vi "子界面-图像预处理.vi"(8 "穿透图":T2(plugin-control)) -> ()   [LabVIEW 2018]
uses:
  <vilib>/vision/NI_Vision_Development_Module.lvlib
panel:
  out "图像分辨率":T1
  in  "stop":bool caption="停止"
  in  "图像预处理":bool
  in  "自定义色彩":bool
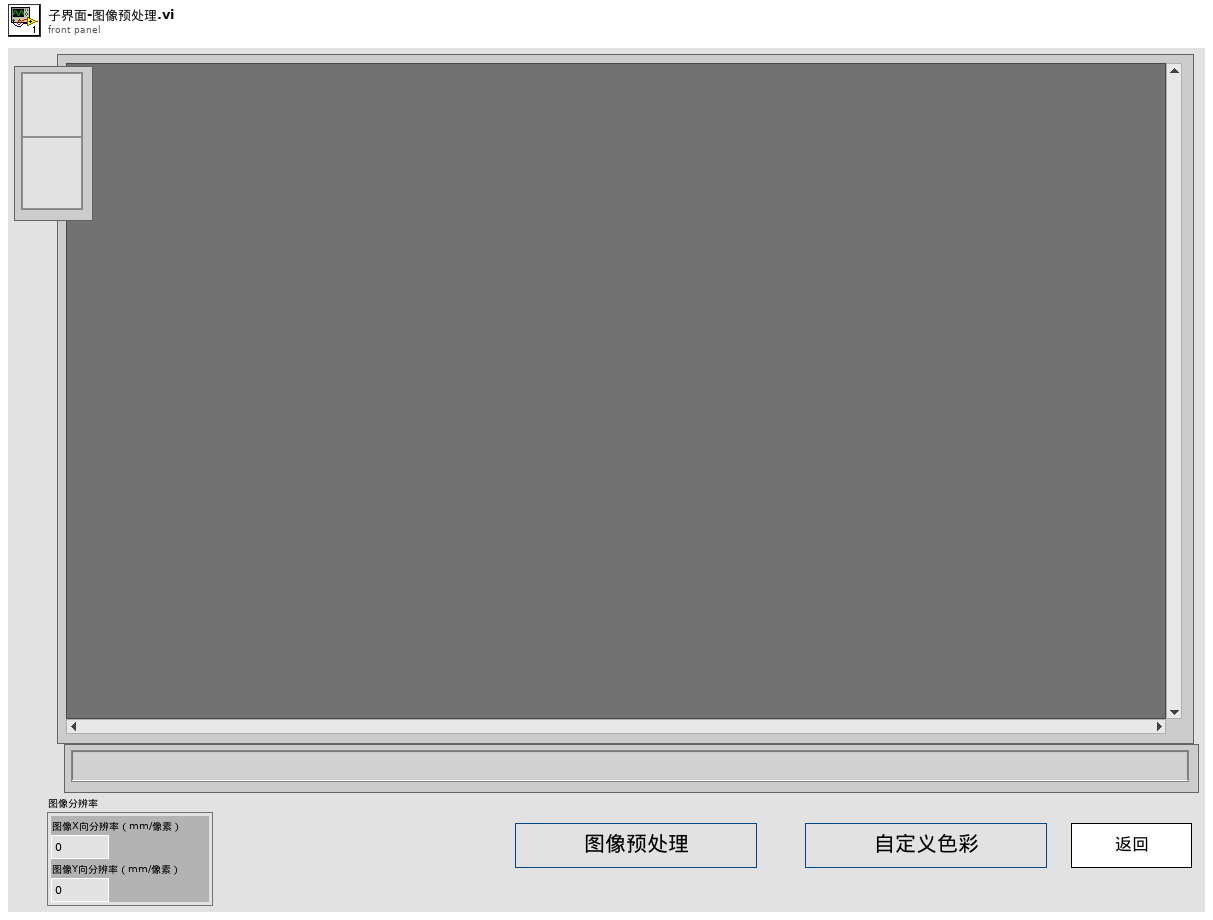
[diagram p1: front panel]
types:
  T1 = cluster{"图像X向分辨率（mm/像素）":dbl, "图像Y向分辨率（mm/像素）":dbl}
  T2 = typedef "IMAQ Image.ctl" = refnum<image>
  T3 = cluster{"Zoom Tool":bool, "Selection Tool":bool, "Pan Tool":bool, "Point Tool":bool, "Line Tool":bool, "Rectangle Tool":bool, "Rotated Rectangle Tool":bool, "Polyline Tool":bool, "Polygon Tool":bool, "Freehand Tool":bool, "Closed Freehand Tool":bool, "Ellipse Tool":bool, "Annulus Tool":bool}
  T4 = enum32{"Linear", "Log", "Exp", "Square", "Square root", "Power X", "Power 1/X"}
  T5 = enum32{"Gray", "Binary", "Gradient", "Rainbow", "Temperature"}
  T6 = enum32{"Invalid", "Standard", "Closed", "Hidden", "Minimized", "Maximized"}
  T7 = cluster{"Red (or Hue) value":u8, "Green (or Sat) value":u8, "Blue (or Light or Val) value":u8}[]
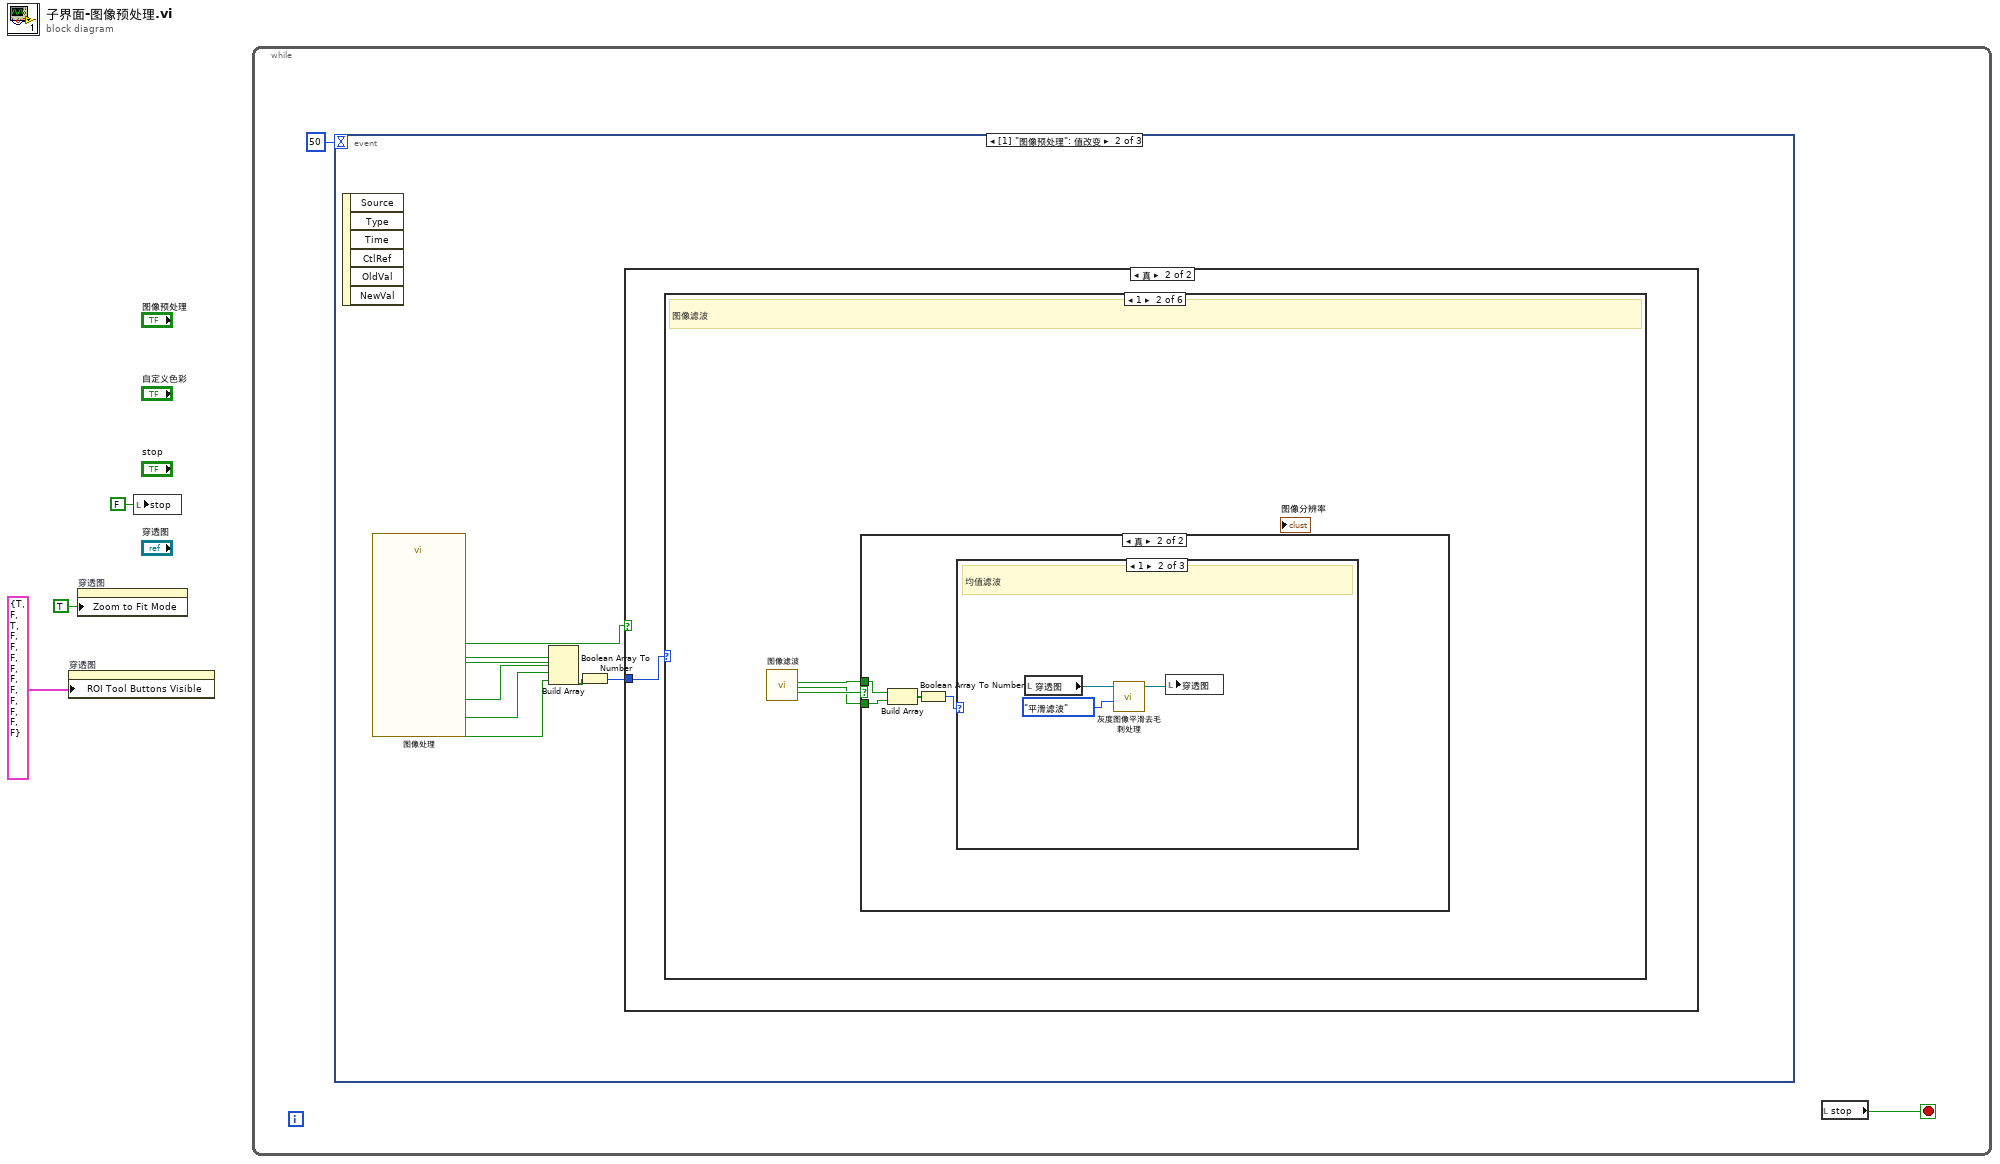
[diagram p0: block diagram]
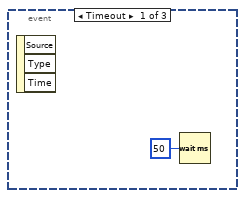
[diagram p2: hidden frame]
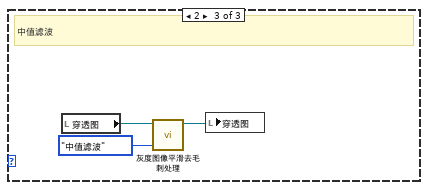
[diagram p7: hidden frame]
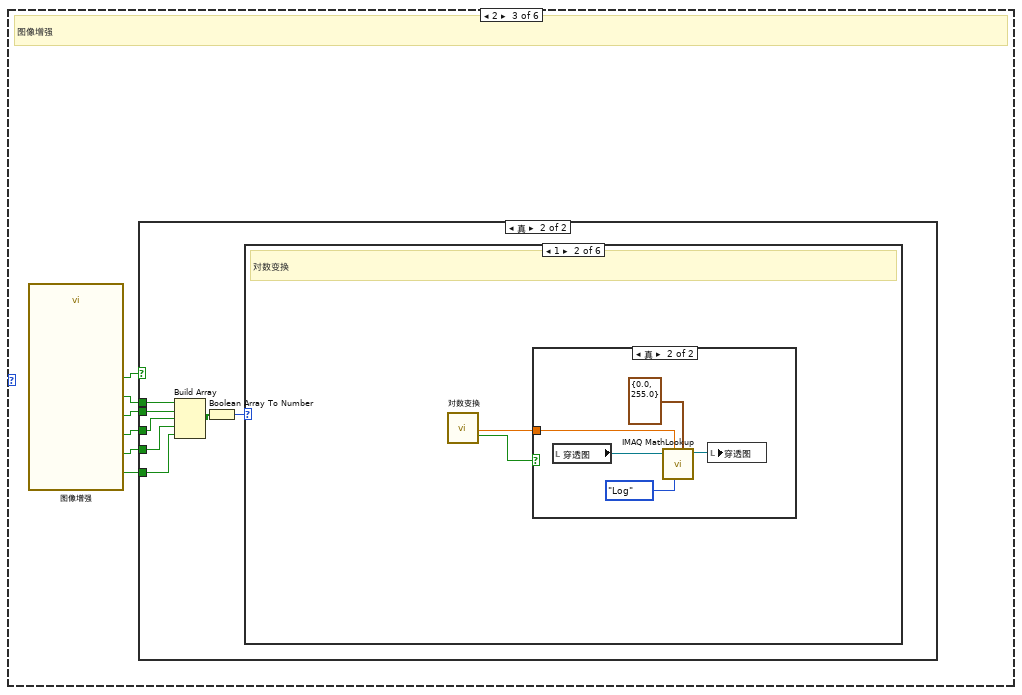
[diagram p8: hidden frame]
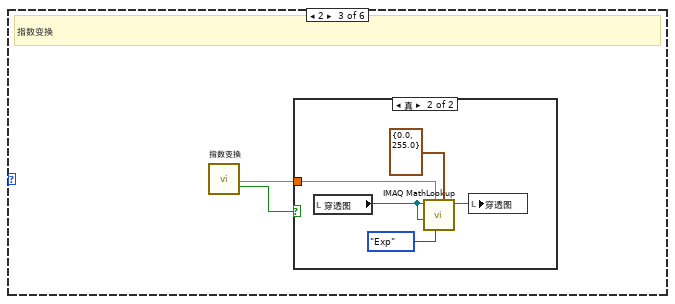
[diagram p12: hidden frame]
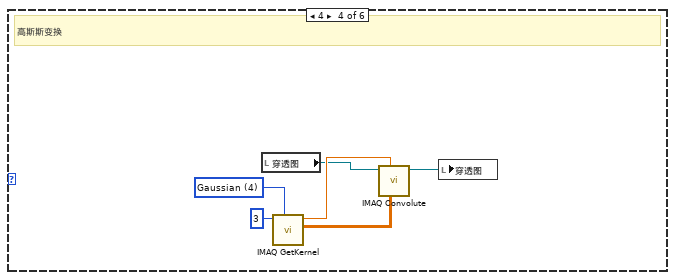
[diagram p14: hidden frame]
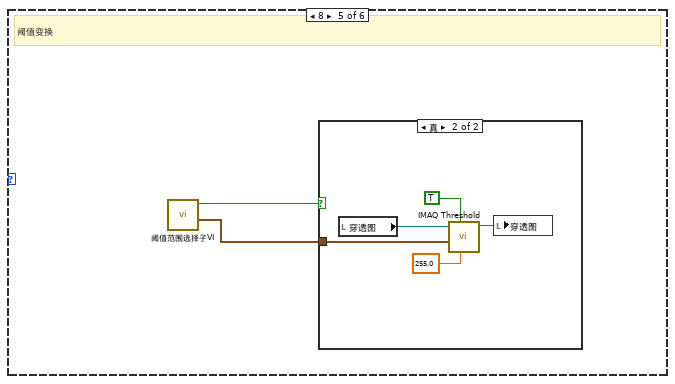
[diagram p15: hidden frame]
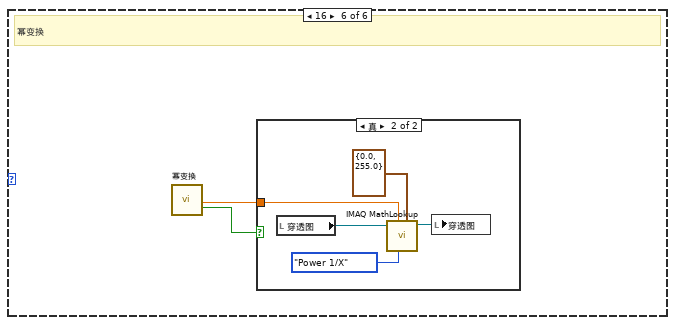
[diagram p17: hidden frame]
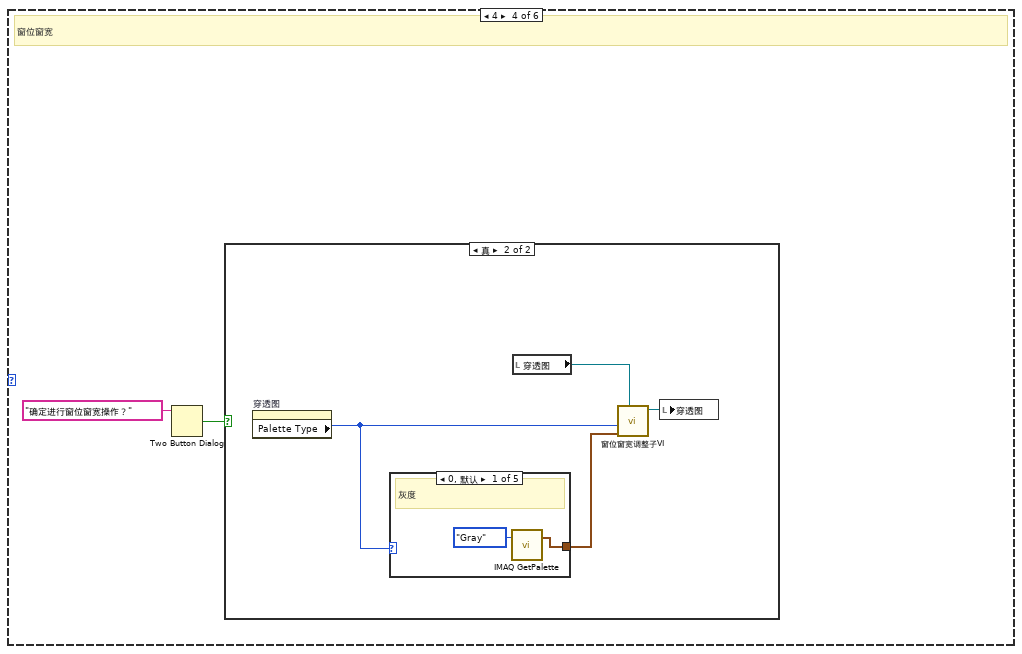
[diagram p19: hidden frame]
diagram:
  n1 = property on="穿透图" class="ImageControl"("ROI Tool Buttons Visible"=T3 {"Zoom Tool"=TRUE, "Selection Tool"=FALSE, "Pan Tool"=TRUE, "Point Tool"=FALSE, "Line Tool"=FALSE, "Rectangle Tool"=FALSE, "Rotated Rectangle Tool"=FALSE, "Polyline Tool"=FALSE, "Polygon Tool"=FALSE, "Freehand Tool"=FALSE, "Closed Freehand Tool"=FALSE, "Ellipse Tool"=FALSE, "Annulus Tool"=FALSE} ("ROI Tool Buttons Visible:All Elements")) -> ()  [unwired: 2 in, 2 out]
  n2 = property on="穿透图" class="ImageControl"("Zoom to Fit Mode"=TRUE) -> ()  [unwired: 2 in, 2 out]
  n3 = local write "stop"(FALSE ("stop")) -> ()
  n4 = while {
    stop <- w5 stop-if-true
    n5 = event shown="[1] \"图像预处理\": 值改变" {
      selector: _ -> [_ _ _]
      dyn-events: _ -> [_ _ _]
      timeout: 50 -> [_ _ _]
      event Timeout {
        n6 = event-data() -> ()  [unwired: 1 in, 3 out]
        n7 = Wait (ms)(milliseconds to wait=u32 50 ("等待时间（毫秒）")) -> ()  [unwired: 1 out]
      }
      event "图像预处理": Value Change {
        n8 = event-data() -> ()  [unwired: 1 in, 6 out]
        n9 = call "图像处理"() -> ("撤销图像处理"=w9:bool, "线性灰度值测量"=w10:bool, "窗位窗宽"=w13:bool, "图像增强"=w11:bool, "图像滤波"=w14:bool, "确定"=w8:bool)  [unwired: 13 in, 1 out]
        n10 = Build Array(w14, w11, w13, w10, w9) -> (w12:bool[])
        n11 = Boolean Array To Number(Boolean array=w12) -> (number=w7:u32)
        n12 = case shown="真" w8 {
          tunnel: w7 -> [_ w15]
          frame False {
          }
          frame True {
            n13 = case shown="1" w15 {
              frame 0, Default {
              }
              frame 1 {
                # "图像滤波"
                n14 = call "图像滤波"() -> ("均值滤波"=w17:bool, "中值滤波"=w16:bool, "确定"=w18:bool)  [unwired: 16 in, 1 out]
                n15 = case shown="真" w18 {
                  tunnel: w17 -> [_ w21]
                  tunnel: w16 -> [_ w20]
                  frame False {
                  }
                  frame True {
                    n16 = Build Array(w21, w20) -> (w22:bool[])
                    n17 = Boolean Array To Number(Boolean array=w22) -> (number=w19:u32)
                    n18 = case shown="1" w19 {
                      frame 0, Default {
                      }
                      frame 1 {
                        # "均值滤波"
                        n19 = local read "穿透图"() -> (w25:T2)
                        n20 = call "灰度图像平滑去毛刺处理.vi"("滤波方法选择"=enum16{"中值滤波", "平滑滤波"}."平滑滤波", "Image"=w25) -> ("Image Out"=w24:T2)  [unwired: 9 in]
                        n21 = local write "穿透图"(w24) -> ()
                      }
                      frame 2 {
                        # "中值滤波"
                        n22 = local read "穿透图"() -> (w28:T2)
                        n23 = call "灰度图像平滑去毛刺处理.vi"("滤波方法选择"=enum16{"中值滤波", "平滑滤波"}."中值滤波", "Image"=w28) -> ("Image Out"=w27:T2)  [unwired: 9 in]
                        n24 = local write "穿透图"(w27) -> ()
                      }
                    }
                  }
                }
              }
              frame 2 {
                # "图像增强"
                n25 = call "图像增强"() -> ("幂变换"=w29:bool, "阈值变换"=w30:bool, "高斯变换"=w31:bool, "指数变换"=w32:bool, "对数变换"=w33:bool, "确定"=w34:bool)  [unwired: 13 in, 1 out]
                n26 = case shown="真" w34 {
                  tunnel: w33 -> [_ w39]
                  tunnel: w32 -> [_ w38]
                  tunnel: w31 -> [_ w37]
                  tunnel: w30 -> [_ w36]
                  tunnel: w29 -> [_ w35]
                  frame False {
                  }
                  frame True {
                    n27 = Build Array(w39, w38, w37, w36, w35) -> (w41:bool[])
                    n28 = Boolean Array To Number(Boolean array=w41) -> (number=w40:u32)
                    n29 = case shown="1" w40 {
                      frame 0, Default {
                      }
                      frame 1 {
                        # "对数变换"
                        n30 = call "对数变换"() -> ("变换系数K"=w42:dbl, "确定"=w43:bool)  [unwired: 17 in, 1 out]
                        n31 = case shown="真" w43 {
                          tunnel: w42 -> [_ w46]
                          frame False {
                          }
                          frame True {
                            n32 = local read "穿透图"() -> (w45:T2)
                            n33 = call "IMAQ MathLookup"("Range"=cluster{"Minimum":sgl, "Maximum":sgl} {"Minimum"=0.0, "Maximum"=255.0}, "Operator"=T4."Log", "X Value"=w46, "Image Src"=w45) -> ("Image Dst Out"=w44:T2)  [unwired: 6 in, 1 out]
                            n34 = local write "穿透图"(w44) -> ()
                          }
                        }
                      }
                      frame 2 {
                        # "指数变换"
                        n35 = call "指数变换"() -> ("变换系数K"=w49:dbl, "确定"=w50:bool)  [unwired: 17 in, 1 out]
                        n36 = case shown="真" w50 {
                          tunnel: w49 -> [_ w51]
                          frame False {
                          }
                          frame True {
                            n37 = local read "穿透图"() -> (w55:T2)
                            n38 = call "IMAQ MathLookup"("Range"=cluster{"Minimum":sgl, "Maximum":sgl} {"Minimum"=0.0, "Maximum"=255.0}, "Operator"=T4."Exp", "X Value"=w51, "Image Dst"=w55, "Image Src"=w55) -> ("Image Dst Out"=w53:T2)  [unwired: 5 in, 1 out]
                            n39 = local write "穿透图"(w53) -> ()
                          }
                        }
                      }
                      frame 4 {
                        w61 = u16 4 items=["Gradient"=1, "Laplacian"=2, "Smoothing"=3, "Gaussian"=4] ("Kernel Family")
                        # "高斯斯变换"
                        n40 = local read "穿透图"() -> (w57:T2)
                        n41 = call "IMAQ GetKernel"("Kernel Family"=w61, "Kernel Size (3,5,...)"=3) -> ("Kernel"=w59:sgl[][], "Divider"=w58:sgl)  [unwired: 6 in, 2 out]
                        n42 = call "IMAQ Convolute"("Kernel"=w59, "Divider (kernel sum)"=w58, "Image Src"=w57) -> ("Image Dst Out"=w56:T2)  [unwired: 7 in, 1 out]
                        n43 = local write "穿透图"(w56) -> ()
                      }
                      frame 8 {
                        # "阈值变换"
                        n44 = call "阈值范围选择子VI.vi"() -> ("阈值范围"=w62:cluster{"Lower value":sgl, "Upper value":sgl}, "确定执行"=w63:bool)  [unwired: 10 in]
                        n45 = case shown="真" w63 {
                          tunnel: w62 -> [_ w67]
                          frame False {
                          }
                          frame True {
                            n46 = local read "穿透图"() -> (w65:T2)
                            n47 = call "IMAQ Threshold"("Replace Value"=sgl 255.0, "Keep/Replace Value (Replace)"=TRUE, "Range"=w67, "Image Src"=w65) -> ("Image Dst Out"=w64:T2)  [unwired: 6 in, 1 out]
                            n48 = local write "穿透图"(w64) -> ()
                          }
                        }
                      }
                      frame 16 {
                        # "幂变换"
                        n49 = call "幂变换"() -> ("变换系数K"=w69:dbl, "确定"=w70:bool)  [unwired: 17 in, 1 out]
                        n50 = case shown="真" w70 {
                          tunnel: w69 -> [_ w73]
                          frame False {
                          }
                          frame True {
                            n51 = local read "穿透图"() -> (w72:T2)
                            n52 = call "IMAQ MathLookup"("Range"=cluster{"Minimum":sgl, "Maximum":sgl} {"Minimum"=0.0, "Maximum"=255.0}, "Operator"=T4."Power 1/X", "X Value"=w73, "Image Src"=w72) -> ("Image Dst Out"=w71:T2)  [unwired: 6 in, 1 out]
                            n53 = local write "穿透图"(w71) -> ()
                          }
                        }
                      }
                    }
                  }
                }
              }
              frame 4 {
                # "窗位窗宽"
                n54 = Two Button Dialog(message="确定进行窗位窗宽操作？" ("消息")) -> (T button?=w77:bool)  [unwired: 2 in]
                n55 = case shown="真" w77 {
                  frame False {
                  }
                  frame True {
                    n56 = property on="穿透图" class="ImageControl"() -> ("Palette Type"=w78:u32)  [unwired: 2 in, 2 out]
                    n57 = case shown="0, 默认" w78 {
                      tunnel: [w82 w84 w86 w88 w90] -> w80
                      frame 0, Default {
                        # "灰度"
                        n58 = call "IMAQ GetPalette"("Palette Number (gray)"=T5."Gray") -> ("Color Palette"=w82:cluster{"Red":u8, "Green":u8, "Blue":u8}[])  [unwired: 4 in, 1 out]
                      }
                      frame 2 {
                        # "梯度"
                        n59 = call "IMAQ GetPalette"("Palette Number (gray)"=T5."Gradient") -> ("Color Palette"=w84:cluster{"Red":u8, "Green":u8, "Blue":u8}[])  [unwired: 4 in, 1 out]
                      }
                      frame 3 {
                        # "彩虹"
                        n60 = call "IMAQ GetPalette"("Palette Number (gray)"=T5."Rainbow") -> ("Color Palette"=w86:cluster{"Red":u8, "Green":u8, "Blue":u8}[])  [unwired: 4 in, 1 out]
                      }
                      frame 4 {
                        # "温度"
                        n61 = call "IMAQ GetPalette"("Palette Number (gray)"=T5."Temperature") -> ("Color Palette"=w88:cluster{"Red":u8, "Green":u8, "Blue":u8}[])  [unwired: 4 in, 1 out]
                      }
                      frame 5 {
                        # "自定义"
                        n62 = property on="穿透图" class="ImageControl"() -> ("User Palette"=w90:cluster{"Red":u8, "Green":u8, "Blue":u8}[])  [unwired: 2 in, 2 out]
                      }
                    }
                    n63 = local read "穿透图"() -> (w79:T2)
                    n64 = call "窗位窗宽调整子VI.vi"("Image in"=w79, "Palette:User Palette"=w80, "Palette:Palette Type"=w78) -> ("Image out"=w81:T2)  [unwired: 8 in]
                    n65 = local write "穿透图"(w81) -> ()
                  }
                }
              }
              frame 8 {
                # "查看线灰度值曲线，用于精确测量"
                n66 = Current VI's Path() -> (path=w97:path)
                n67 = Open VI Reference(vi path=w97) -> (vi reference=w96:refnum<vi>, error out=w94:errorcluster)  [unwired: 5 in]
                n68 = property class="VI"(reference=w96, error in=w94, "FP.State"=T6."Hidden" ("前面板窗口:状态")) -> (reference out=w95:refnum<vi>, error out=w93:errorcluster)
                n69 = Close Reference(reference=w95, error in (no error)=w93) -> (error out=w91:errorcluster)
                n70 = case shown="无错误" w91 {
                  frame No Error {
                    n71 = property on="穿透图" class="ImageControl"() -> ("Palette Type"=w98:u32)  [unwired: 2 in, 2 out]
                    n72 = case shown="5" w98 {
                      tunnel: [w102 w104 w106 w108 w110] -> w100
                      frame 0, Default {
                        # "灰度"
                        n73 = call "IMAQ GetPalette"("Palette Number (gray)"=T5."Gray") -> ("Color Palette"=w102:cluster{"Red":u8, "Green":u8, "Blue":u8}[])  [unwired: 4 in, 1 out]
                      }
                      frame 2 {
                        # "梯度"
                        n74 = call "IMAQ GetPalette"("Palette Number (gray)"=T5."Gradient") -> ("Color Palette"=w104:cluster{"Red":u8, "Green":u8, "Blue":u8}[])  [unwired: 4 in, 1 out]
                      }
                      frame 3 {
                        # "彩虹"
                        n75 = call "IMAQ GetPalette"("Palette Number (gray)"=T5."Rainbow") -> ("Color Palette"=w106:cluster{"Red":u8, "Green":u8, "Blue":u8}[])  [unwired: 4 in, 1 out]
                      }
                      frame 4 {
                        # "温度"
                        n76 = call "IMAQ GetPalette"("Palette Number (gray)"=T5."Temperature") -> ("Color Palette"=w108:cluster{"Red":u8, "Green":u8, "Blue":u8}[])  [unwired: 4 in, 1 out]
                      }
                      frame 5 {
                        # "自定义"
                        n77 = property on="穿透图" class="ImageControl"() -> ("User Palette"=w110:cluster{"Red":u8, "Green":u8, "Blue":u8}[])  [unwired: 2 in, 2 out]
                      }
                    }
                    n78 = local read "穿透图"() -> (w99:T2)
                    n79 = local read "图像分辨率"() -> (w101:T1)
                    n80 = call "线性灰度值曲线查看子VI.vi"("Palette:User Palette"=w100, "图像分辨率"=w101, "Image"=w99) -> ()  [unwired: 9 in]
                  }
                  frame Error {
                  }
                }
              }
              frame 16 {
                # "撤销图像处理，恢复原图"
                n81 = call "IMAQ Create"("Image Name"="P1") -> ("New Image"=w111:T2)  [unwired: 4 in, 1 out]
                n82 = local write "穿透图"(w111) -> ()
              }
            }
          }
        }
      }
      event "自定义色彩": Value Change {
        n83 = event-data() -> ()  [unwired: 1 in, 6 out]
        n84 = call "调色板"() -> ("自定义显示"=w118:bool, "温度显示"=w117:bool, "彩虹显示"=w116:bool, "梯度显示"=w115:bool, "灰度显示"=w114:bool, "确定"=w113:bool)  [unwired: 13 in, 1 out]
        n85 = Build Array(w114, w115, w116, w117, w118) -> (w119:bool[])
        n86 = case shown="真" w113 {
          tunnel: w119 -> [_ w122]
          frame False {
          }
          frame True {
            n87 = Boolean Array To Number(Boolean array=w122) -> (number=w121:u32)
            n88 = case shown="16" w121 {
              tunnel: [w123 w124 w125 w126 w127 w129] -> w120
              frame 0, Default {
                w123 = u32 0 items=["Grayscale", "Binary", "Gradient", "Rainbow", "Temperature", "User Defined", "Binary 16 Bit", "Gradient 16 Bit", "Rainbow 16 Bit", "Temperature 16 Bit", "User Defined 16 Bit"] ("Palette:Palette Type")
              }
              frame 1 {
                w124 = u32 0 items=["Grayscale", "Binary", "Gradient", "Rainbow", "Temperature", "User Defined", "Binary 16 Bit", "Gradient 16 Bit", "Rainbow 16 Bit", "Temperature 16 Bit", "User Defined 16 Bit"] ("Palette:Palette Type")
                # "灰度"
              }
              frame 2 {
                w125 = u32 2 items=["Grayscale", "Binary", "Gradient", "Rainbow", "Temperature", "User Defined", "Binary 16 Bit", "Gradient 16 Bit", "Rainbow 16 Bit", "Temperature 16 Bit", "User Defined 16 Bit"] ("Palette:Palette Type")
                # "梯度"
              }
              frame 4 {
                w126 = u32 3 items=["Grayscale", "Binary", "Gradient", "Rainbow", "Temperature", "User Defined", "Binary 16 Bit", "Gradient 16 Bit", "Rainbow 16 Bit", "Temperature 16 Bit", "User Defined 16 Bit"] ("Palette:Palette Type")
                # "彩虹"
              }
              frame 8 {
                w127 = u32 4 items=["Grayscale", "Binary", "Gradient", "Rainbow", "Temperature", "User Defined", "Binary 16 Bit", "Gradient 16 Bit", "Rainbow 16 Bit", "Temperature 16 Bit", "User Defined 16 Bit"] ("Palette:Palette Type")
                # "温度"
              }
              frame 16 {
                w129 = u32 5 items=["Grayscale", "Binary", "Gradient", "Rainbow", "Temperature", "User Defined", "Binary 16 Bit", "Gradient 16 Bit", "Rainbow 16 Bit", "Temperature 16 Bit", "User Defined 16 Bit"] ("Palette:Palette Type")
                # "自定义"
                n89 = call "自定义成像色谱20200214.vi"() -> ("Color palette"=w128:T7)  [unwired: 8 in, 1 out]
                n90 = property on="穿透图" class="ImageControl"("User Palette"=w128) -> ()  [unwired: 2 in, 2 out]
              }
            }
            n91 = property on="穿透图" class="ImageControl"("Palette Type"=w120) -> ()  [unwired: 2 in, 2 out]
          }
        }
      }
    }
    n92 = local read "stop"() -> (w5:bool)
  }
